vi "이미지 데이터 셋 저장.vi"() -> ()   [LabVIEW 2020]
uses:
  <vilib>/userDefined/High Color/IMAQdx.ctl
  <vilib>/vision/driver/NI_Vision_Acquisition_Software.lvlib
panel:
  out "현재 개수":string
  in  "시작 개수":string="0"
  in  "저장 경로":path
  out "Capture Image":T1(plugin-control)
  in  "확인 버튼":bool
  out "Image":T1(plugin-control)
  in  "정지":bool
  # "1조부터 4조까지 데이터셋을 모으는데,\n\n1조는 0부터 시작\n2조는 10000부터 시작\n3조는 20000부터 시작\n4조는 30000부터 시작\n\n으로 해주시기 바랍니다.\n\n데이터셋이 다 모이면 취합 예정"
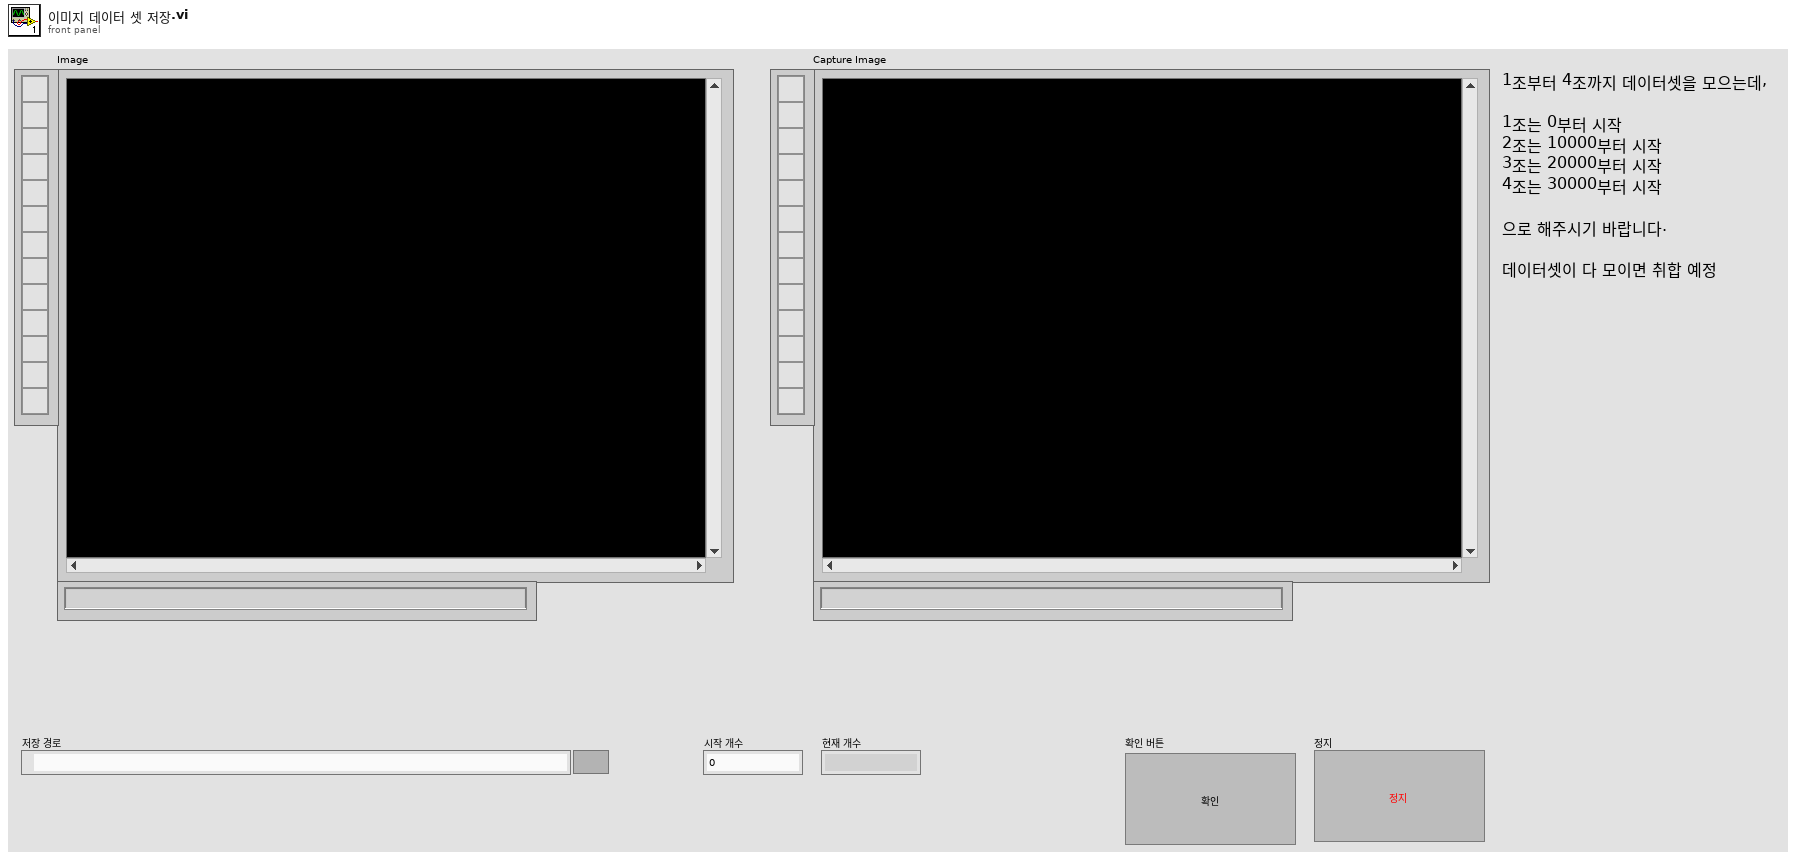
[diagram p1: front panel]
types:
  T1 = typedef "IMAQ Image.ctl" = refnum<image>
  T2 = typedef "Image Type" = u32
  T3 = typedef "IMAQdx.ctl" = refnum<k21>
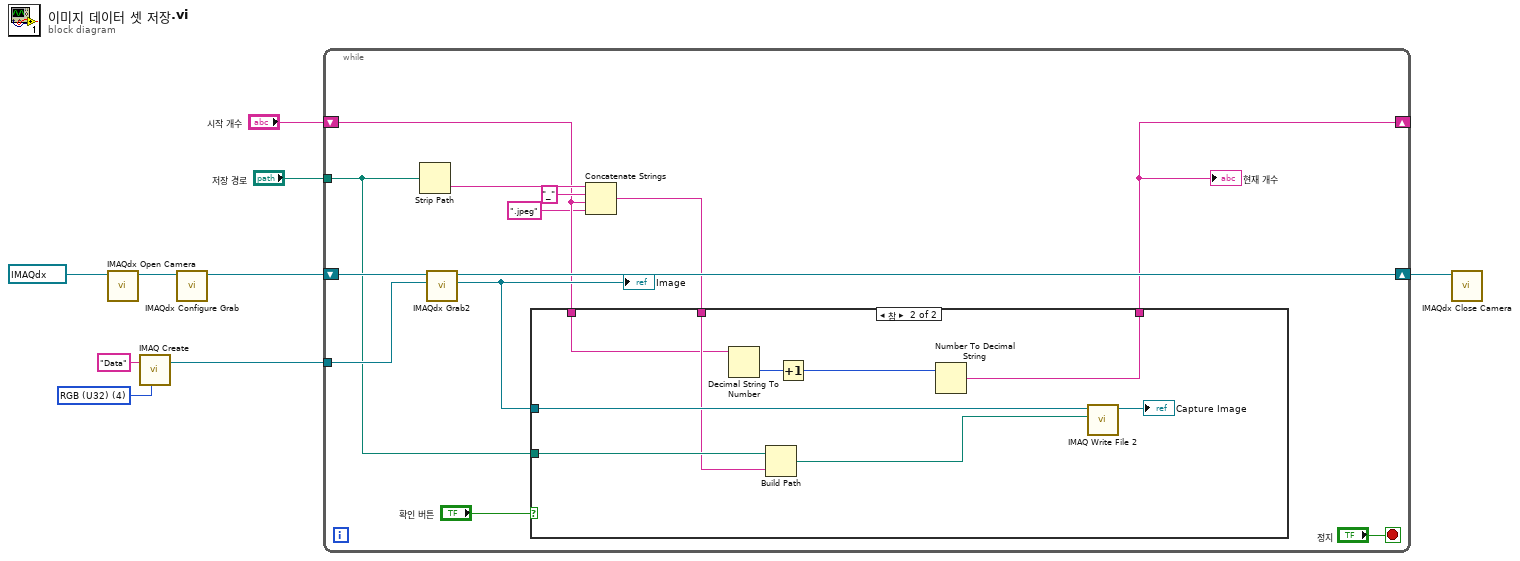
[diagram p0: block diagram]
diagram:
  w4 = T2 4 items=["Grayscale (U8)", "Grayscale (I16)", "Grayscale (SGL)", "Complex (CSG)", "RGB (U32)", "HSL (U32)", "RGB (U64)", "Grayscale (U16)"] ("Image Type")
  n1 = call <vilib>:"IMAQdx Open Camera.vi"("Session In"=T3 "cam2") -> ("Session Out"=w8:T3)  [unwired: 9 in, 1 out]
  n2 = call "IMAQ Create"("Image Name"="Data", "Image Type"=w4) -> ("New Image"=w3:T1)  [unwired: 3 in, 1 out]
  n3 = call <vilib>:"IMAQdx Configure Grab.vi"("Session In"=w8) -> ("Session Out"=w7:T3)  [unwired: 9 in, 1 out]
  n4 = while {
    shift-right: [w20] -> w6
    shift-left: w7 -> [w21]
    tunnel: w3 -> [w19]
    tunnel: "저장 경로" -> [w14]
    shift-right: [w10] -> _
    shift-left: "시작 개수" -> [w12]
    stop <- "정지" stop-if-true
    n5 = Strip Path(path=w14) -> (name=w16:string)  [unwired: 1 out]
    n6 = call <vilib>:"IMAQdx Grab2.vi"("Image In"=w19, "Session In"=w21) -> ("Image Out"=w17:T1, "Session Out"=w20:T3)  [unwired: 6 in, 2 out]
    "Image" <- w17
    n7 = Concatenate Strings(w16, "_" ("문자열"), w12, ".jpeg" ("문자열")) -> (w13:string)
    n8 = case shown="참" "확인 버튼" {
      tunnel: w17 -> [_ w32]
      tunnel: w14 -> [_ w30]
      tunnel: w13 -> [_ w29]
      tunnel: w12 -> [w23 w27]
      tunnel: [w23 w24] -> w10
      frame False {
      }
      frame True {
        n9 = Decimal String To Number(string=w27) -> (number=w26:i32)  [unwired: 2 in, 1 out]
        n10 = Build Path(base path=w30, name or relative path=w29) -> (appended path=w28:path)
        n11 = Increment(x=w26) -> (x+1=w25:i32)
        n12 = Number To Decimal String(number=w25) -> (decimal integer string=w24:string)  [unwired: 1 in]
        n13 = call-poly "IMAQ Write File 2"("File Path"=w28, "Image"=w32) -> ("Image Out (duplicate)"=→"Capture Image":T1)  [unwired: 8 in, 1 out]
      }
    }
    "현재 개수" <- w10
  }
  n14 = call <vilib>:"IMAQdx Close Camera.vi"("Session In"=w6) -> ()  [unwired: 10 in, 1 out]
